vi "Análise de Temperatura.vi"() -> ()   [LabVIEW 2021]
uses:
  <vilib>/Analysis/NI_AALBase.lvlib
  <vilib>/Analysis/NI_AALPro.lvlib
panel:
  out "Polynomial Coefficients":dbl[](array[numeric]) format="%#.2g"
  out "Waveform Graph":cluster{i32, dbl, "Best Polynomial Fit":dbl[]}[](graph)
  in  "polynomial order":i32=2
  out "variance":dbl format="%.2f"
  out "standard deviation":dbl format="%.2f"
  out "mean":dbl format="%.2f"
  out "min value":dbl format="%#.2g"
  out "max value":dbl format="%#.2g"
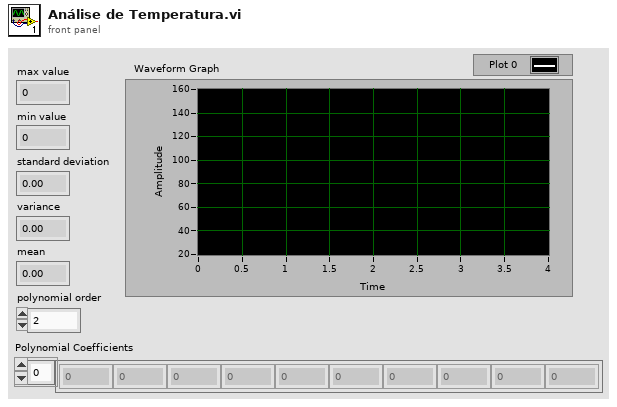
[diagram p1: front panel]
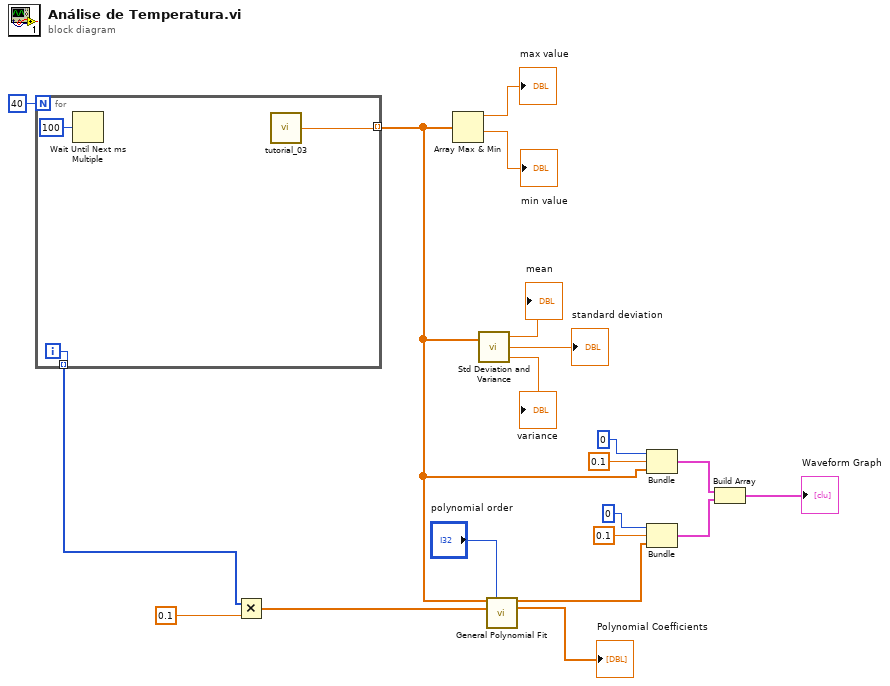
[diagram p0: block diagram]
diagram:
  n1 = for {
    N: 40 -> [_]
    tunnel: [w22] -> w8 mode=indexing
    tunnel: [w21] -> w14 mode=indexing
    i -> [w21]
    n2 = Wait Until Next ms Multiple(millisecond multiple=u32 100) -> ()  [unwired: 1 out]
    n3 = call "tutorial_03.vi"() -> ("Thermometer"=w22:dbl)  [unwired: 2 in]
  }
  n4 = Multiply(x=w14, y=0.1) -> (x*y=w13:dbl[])
  n5 = Array Max & Min(array=w8) -> (max value=→"max value":dbl, min value=→"min value":dbl)  [unwired: 2 out]
  n6 = call <vilib>:"Std Deviation and Variance.vi"("X"=w8) -> ("mean"=→"mean":dbl, "standard deviation"=→"standard deviation":dbl, "variance"=→"variance":dbl)  [unwired: 1 in]
  n7 = call <vilib>:"General Polynomial Fit.vi"("Y"=w8, "polynomial order"="polynomial order", "X"=w13) -> ("Best Polynomial Fit"=w5:dbl[], "Polynomial Coefficients"=→"Polynomial Coefficients":dbl[])  [unwired: 9 in, 2 out]
  n8 = Bundle(0, 0.1, w8) -> (w4:cluster{i32, dbl, dbl[]})  [unwired: 1 in]
  n9 = Bundle(0, 0.1, "Best Polynomial Fit"=w5) -> (w3:cluster{i32, dbl, "Best Polynomial Fit":dbl[]})  [unwired: 1 in]
  n10 = Build Array(w4, w3) -> (→"Waveform Graph":cluster{i32, dbl, "Best Polynomial Fit":dbl[]}[])
